vi "runAScript.vi"(10 "Path":string="\\\\Zeus\\C$\\Documents and Settings\\Administrator\\Desktop\\Crete\\Data\\Scripts\\ScriptRunFolder\\Dipole Trap Script_v2.xml") -> (1 "stoppedByUser":bool, 2 "TimeStamp":string)   [LabVIEW 2011, in "run.lvlib"]
uses:
  run.lvlib
  Viewers/Editors/ExperimentRunner/Events/ExperimentControlEvents.lvclass
  Viewers/ExperimentControl.lvlib
  Events/Event.lvclass
  Tools/Filing/FileNeologist/FileNeologist.lvclass
  Tools/Filing.lvlib
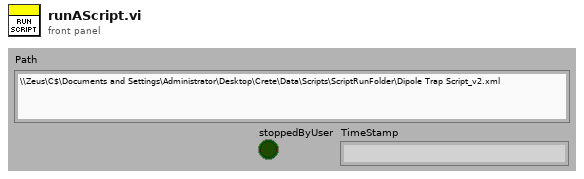
[diagram p1: front panel]
types:
  T1 = enum16{"close", "stopRunning", "runSingleScript", "runExperiment", "runExperimentScript", "Unregistered", "hasStopped"}
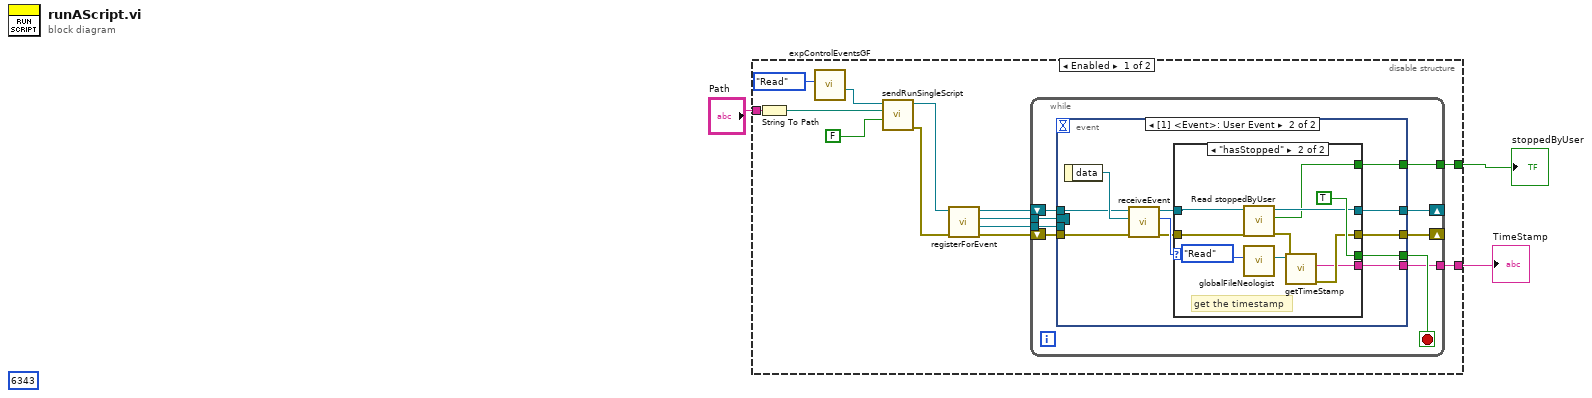
[diagram p0: block diagram]
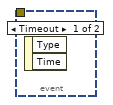
[diagram p2: hidden frame]
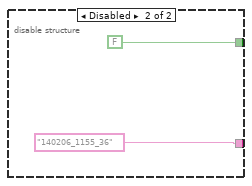
[diagram p4: hidden frame]
diagram:
  (unwired) 6343
  n1 = disable-structure shown="Enabled" {
    disable-tunnel: "Path" -> [w16 _]
    disable-tunnel: [w5 "140206_1155_36"] -> w2
    disable-tunnel: [w4 FALSE] -> w1
    frame Enabled {
      n2 = String To Path(string=w16) -> (path=w14:path)
      n3 = call "expControlEventsGF.vi"("Action"=enum16{"Write", "Read"}."Read") -> ("ExperimentControlEvents"=w13:refnum<class "ExperimentControlEvents.lvclass">)  [unwired: 10 in]
      n4 = call "sendRunSingleScript.vi"("HWLoop"=FALSE, "Path"=w14, "ExperimentControlEvents in"=w13) -> ("error out"=w11:errorcluster, "ExperimentControlEvents out"=w10:refnum<class "ExperimentControlEvents.lvclass">)  [unwired: 7 in]
      n5 = call "registerForEvent.vi"("error in (no error)"=w11, "Event in"=w10) -> ("error out"=w6:errorcluster, "Event"=w8:refnum<user-event>, "Event Registration Refnum"=w9:refnum<event-registration>, "Event out"=w7:refnum<class "ExperimentControlEvents.lvclass">)  [unwired: 6 in]
      n6 = while {
        tunnel: w9 -> [w25]
        tunnel: w8 -> [w24]
        shift-right: [w21] -> _
        shift-left: w7 -> [w23]
        shift-right: [w20] -> _
        shift-left: w6 -> [w22]
        tunnel: [w18] -> w5
        tunnel: [w17] -> w4
        stop <- w19 stop-if-true
        n7 = event shown="[1] <Event>: User Event" {
          selector: w25 -> [_ _]
          dyn-events: _ -> [_ _]
          timeout: _ -> [_ _]
          tunnel: w24 -> [_ _]
          tunnel: w23 -> [_ w35]
          tunnel: w22 -> [_ w34]
          tunnel: [_ w30] -> w21
          tunnel: [_ w31] -> w20
          tunnel: [_ w28] -> w19
          tunnel: [_ w27] -> w18
          tunnel: [_ w26] -> w17
          event Timeout {
            n8 = event-data() -> ()  [unwired: 1 in, 2 out]
          }
          event User Event {
            n9 = event-data() -> ("data"=w36:refnum<class>)  [unwired: 1 in]
            n10 = call "receiveEvent.vi"("error in (no error)"=w34, "data"=w36, "ExperimentControlEvents in"=w35) -> ("error out"=w32:errorcluster, "Enum"=w33:T1, "ExperimentControlEvents out"=w29:refnum<class "ExperimentControlEvents.lvclass">)  [unwired: 6 in]
            n11 = case shown="\"hasStopped\"" w33 {
              tunnel: w32 -> [w37 w42]
              tunnel: [w37 w45] -> w31
              tunnel: [w38 w40] -> w30
              tunnel: w29 -> [w38 w43]
              tunnel: [_ TRUE] -> w28
              tunnel: [_ w44] -> w27
              tunnel: [_ w39] -> w26
              frame Default {
              }
              frame "hasStopped" {
                # "get the timestamp"
                n12 = call "Read stoppedByUser.vi"("error in (no error)"=w42, "ExperimentControlEvents in"=w43) -> ("error out"=w41:errorcluster, "stoppedByUser"=w39:bool, "ExperimentControlEvents out"=w40:refnum<class "ExperimentControlEvents.lvclass">)  [unwired: 7 in]
                n13 = call "globalFileNeologist.vi"("Action"=enum16{"Write", "Read"}."Read") -> ("FileNeologist out"=w46:refnum<class "FileNeologist.lvclass">)  [unwired: 10 in]
                n14 = call "getTimeStamp.vi"("error in (no error)"=w41, "FileNeologist in"=w46) -> ("error out"=w45:errorcluster, "TimeStamp"=w44:string)  [unwired: 7 in, 1 out]
              }
            }
          }
        }
      }
    }
    frame Disabled {
    }
  }
  "TimeStamp" <- w2
  "stoppedByUser" <- w1
